vi "GF_SortWavesWithNameArray.vi"(2 "WaveNames In":string[](array[string]), 3 "WaveformData In":waveform(dbl)[](array[waveform])) -> (0 "WaveNames Out":string[](array[string]), 1 "WaveformData Out":waveform(dbl)[](array[waveform]))   [LabVIEW 2016]
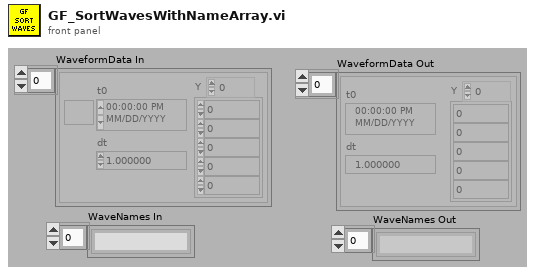
[diagram p1: front panel]
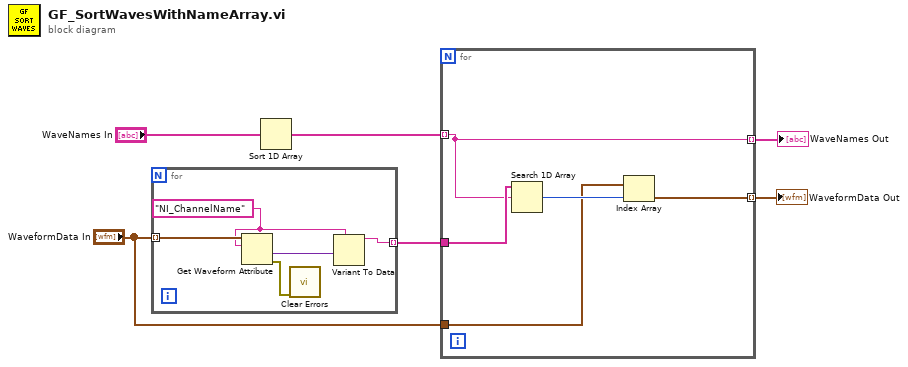
[diagram p0: block diagram]
diagram:
  n1 = for {
    tunnel: "WaveformData In" -> [w11] mode=indexing
    tunnel: [w7] -> w4 mode=indexing
    w8 = "NI_ChannelName" ("name")
    n2 = Get Waveform Attribute(6:w8, 7:w11) -> (0:w10:errorcluster, 1:w9:variant)  [unwired: 2 in, 2 out]
    n3 = call <vilib>:"Clear Errors.vi"("error in (no error)"=w10) -> ()  [unwired: 5 in, 2 out]
    n4 = Variant To Data(type=w8, Variant=w9) -> (data=w7:string)  [unwired: 1 in, 1 out]
  }
  n5 = Sort 1D Array(array="WaveNames In") -> (sorted array=w5:string[])
  n6 = for {
    tunnel: w5 -> [w13] mode=indexing
    tunnel: w4 -> [w16]
    tunnel: "WaveformData In" -> [w14]
    tunnel: [w13] -> w2 mode=indexing
    tunnel: [w12] -> w1 mode=indexing
    n7 = Search 1D Array(1D array=w16, element=w13) -> (index of element=w15:i32)  [unwired: 1 in]
    n8 = Index Array(array=w14, index=w15) -> (element=w12:waveform(dbl))
  }
  "WaveformData Out" <- w1
  "WaveNames Out" <- w2
